vi "Update VeriStand Channel Values.vi"(6 "SignalIds Out":i32[](array[numeric]), 7 "SignalIds In":i32[](array[numeric]), 8 "error in":errorcluster, 10 "Write Ref":T2, 11 "Read Write Ref":T1) -> (0 "error out":errorcluster)   [LabVIEW 2026, in "Runtime Configuration Support Inline Async Example Custom Device Engine.lvlib"]
uses:
  Runtime Configuration Support Inline Async Example Custom Device Engine.lvlib
  <vilib>/NI/NIVS Inline Async API/_Data Access Engine/Data Access Engine/Types/Write.DVR.ctl
  <vilib>/NI/NIVS Inline Async API/_Data Access Engine/Access Type Classes/Write/Write.lvclass
  <vilib>/NI/NIVS Inline Async API/_Data Access Engine/Data Access Engine/Types/ReadWrite.DVR.ctl
  <vilib>/NI/NIVS Inline Async API/_Data Access Engine/Access Type Classes/ReadWrite/ReadWrite.lvclass
  <vilib>/NI/NIVS Inline Async API/_Data Access Engine/Access Type Classes/Write/Write.lvclass/Write.ctl
  <vilib>/NI/NIVS Inline Async API/_Data Access Engine/Access Type Classes/ReadWrite/ReadWrite.lvclass/ReadWrite.ctl
  <vilib>/NI/NIVS Inline Async API/_Data Access Engine/Data Access Engine/Methods/Write.Data.vi
  <vilib>/NI/NIVS Inline Async API/_Data Access Engine/Data Access Engine/Methods/ReadWrite.Data.Write.vi
  <vilib>/NI/NIVS Inline Async API/_Data Access Engine/Access Type Classes/Write/Write.ProcessData.vi
  <vilib>/NI/NIVS Inline Async API/_Data Access Engine/Access Type Classes/ReadWrite/ReadWrite.ProcessData.Write.vi
  <vilib>/NI/NIVS Inline Async API/_Data Access Engine/Access Type Classes/ReadWrite/ReadWrite.EngineData.vi
  <vilib>/NI/NIVS Inline Async API/_Data Access Engine/Access Type Classes/Write/Write.Buffer.vi
  <vilib>/NI/NIVS Inline Async API/_Data Access Engine/Access Type Classes/Write/Write.Commit.vi
  <vilib>/NI/NIVS Inline Async API/_Data Access Engine/Access Type Classes/ReadWrite/ReadWrite.ProcessData.Buffer.vi
  <vilib>/NI/NIVS Inline Async API/_Data Access Engine/Access Type Classes/ReadWrite/ReadWrite.ProcessData.Commit.vi
  <vilib>/NI VeriStand/Custom Device API/NI VeriStand - Get Channel Value by Data Reference.vi
  <vilib>/NI VeriStand/Custom Device API/NI VeriStand - Set Channel Value by Data Reference.vi
  <vilib>/NI VeriStand/Custom Device API/Global Data Refs.vi
  <vilib>/NI/NIVS Inline Async API/_Data Access Engine/Data Access Engine/Data Access Engine.lvclass
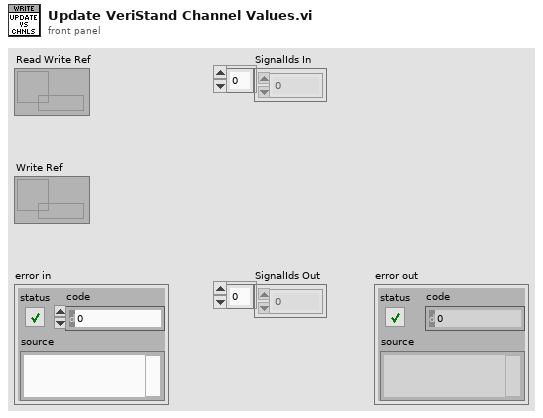
[diagram p1: front panel]
types:
  T1 = typedef "Data Access Engine.lvlib/Data Access Engine.lvclass/ReadWrite.DVR.ctl" = refnum<data-value>
  T2 = typedef "Data Access Engine.lvlib/Data Access Engine.lvclass/Write.DVR.ctl" = refnum<data-value>
  T3 = enum16{"Initialize", "Set In Val", "Get In Val", "Set Block", "Set Out Val", "Get Out Val", "Get In Array", "Get Out Array"}
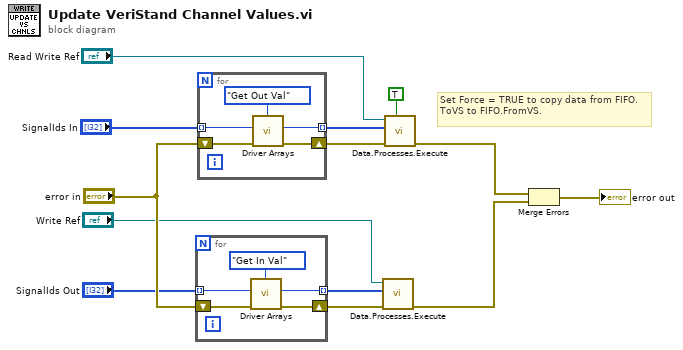
[diagram p0: block diagram]
diagram:
  # "Set Force = TRUE to copy data from FIFO.ToVS to FIFO.FromVS."
  n1 = for {
    tunnel: "SignalIds Out" -> [w16] mode=indexing
    tunnel: [w14] -> w3 mode=indexing
    shift-right: [w18] -> w12
    shift-left: "error in" -> [w17]
    n2 = call "Driver Arrays.vi"("error in"=w17, "Index"=w16, "Curr Operation"=T3."Get In Val") -> ("error out"=w18:errorcluster, "Value"=w14:i32)  [unwired: 5 in, 2 out]
  }
  n3 = for {
    tunnel: "SignalIds In" -> [w21] mode=indexing
    tunnel: [w19] -> w4 mode=indexing
    shift-right: [w23] -> w13
    shift-left: "error in" -> [w22]
    n4 = call "Driver Arrays.vi"("error in"=w22, "Index"=w21, "Curr Operation"=T3."Get Out Val") -> ("error out"=w23:errorcluster, "Value"=w19:i32)  [unwired: 5 in, 2 out]
  }
  n5 = call-poly <vilib>:"Data.Processes.Execute.vi"("error in (no error)"=w12, "Values"=w3, "Ref"="Write Ref") -> ("error out"=w9:errorcluster)  [unwired: 8 in]
  n6 = call-poly <vilib>:"Data.Processes.Execute.vi"("Force"=TRUE, "error in"=w13, "Values"=w4, "Ref"="Read Write Ref") -> ("error out"=w10:errorcluster)  [unwired: 7 in]
  n7 = Merge Errors(w10, w9) -> (→"error out":errorcluster)
